vi "svfa_Window Frequency Response.vi"   [LabVIEW 2017]
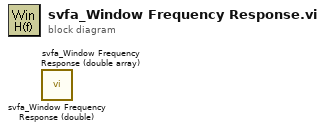
[diagram p0: block diagram]
diagram:
  n1 = call <vilib>:"svfa_Window Frequency Response (double).vi"() -> ()  [unwired: 3 in, 1 out]
  n2 = call <vilib>:"svfa_Window Frequency Response (double array).vi"() -> ()  [unwired: 3 in, 1 out]
